vi "Get Desired Size.vi"(8 "error in (no error)":errorcluster, 11 "ColumnPanel in":refnum<class "ColumnPanel.lvclass">) -> (0 "error out":errorcluster, 2 "Desired Size":T1, 3 "ColumnPanel out":refnum<class "ColumnPanel.lvclass">)   [LabVIEW 2020, in "Conditum-Tools.lvlib" / "ColumnPanel.lvclass"]
uses:
  ColumnPanel.lvclass
  <vilib>/IlluminatedG/IG OOPanel/OOPanel/ArrayPanel/Desired Size.ctl
  ColumnPanel.lvclass/ColumnPanel.ctl
  <vilib>/IlluminatedG/IG OOPanel/OOPanel/OOPanel.lvlib
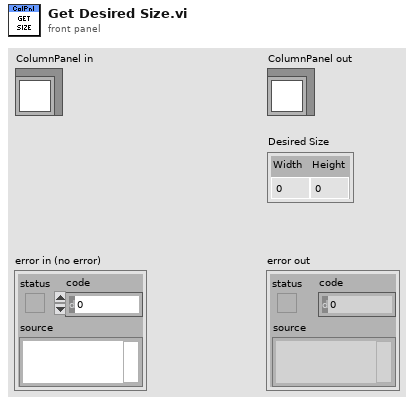
[diagram p1: front panel]
types:
  T1 = typedef "OOPanel.lvlib/Desired Size.ctl" = cluster{"Width":u32, "Height":u32}
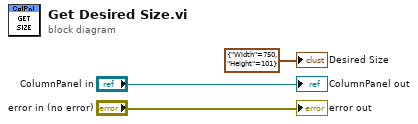
[diagram p0: block diagram]
diagram:
  "error out" <- "error in (no error)"
  "ColumnPanel out" <- "ColumnPanel in"
  "Desired Size" <- T1 {"Width"=750, "Height"=101} ("Desired Size")
